vi "Signal Express Vi.vi"() -> ()   [LabVIEW 2022 SP3]
panel:
  in  "Frequency":dbl=10.1
  in  "stop":bool
  out "Waveform Graph":dynamicdata(graph)
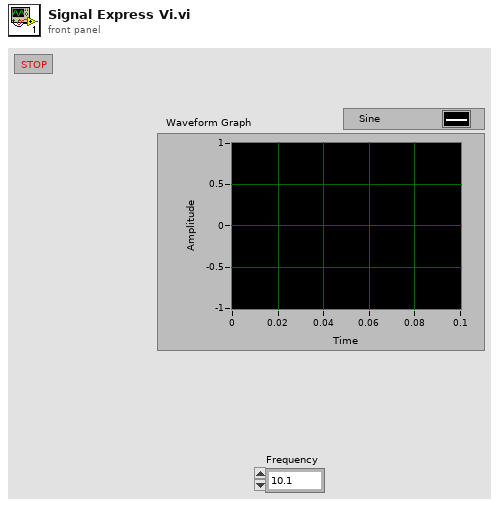
[diagram p1: front panel]
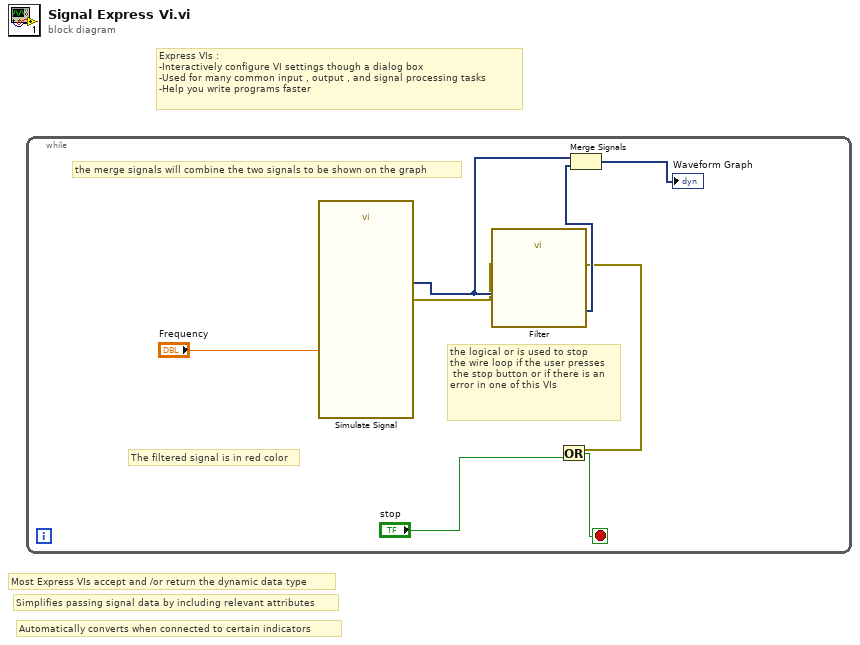
[diagram p0: block diagram]
diagram:
  # "Automatically converts when connected to certain indicators"
  # "Simplifies passing signal data by including relevant attributes"
  # "Most Express VIs accept and /or return the dynamic data type"
  # "Express VIs :\n-Interactively configure VI settings though a dialog box\n-Used for many common input , output , and signal processing tasks\n-Help you write programs faster"
  n1 = while {
    stop <- w7 stop-if-true
    # "The filtered signal is in red color"
    # "the logical or is used to stop\nthe wire loop if the user presses\n the stop button or if there is an \nerror in one of this VIs"
    # "the merge signals will combine the two signals to be shown on the graph"
    n2 = call "Simulate Signal"("Frequency"="Frequency") -> ("Sine"=w6:dynamicdata, "error out"=w3:errorcluster)  [unwired: 13 in]
    n3 = call "Filter"("error in (no error)"=w3, "Signal"=w6) -> ("error out"=w2:errorcluster, "Filtered Signal"=w5:dynamicdata)  [unwired: 8 in]
    n4 = Or(x=w2, y="stop") -> (x .or. y?=w7:bool)
    n5 = Merge Signals(w6, w5) -> (→"Waveform Graph":dynamicdata)
  }
